vi "RIOduino Periodic.vi"   [LabVIEW 2015]
uses:
  <vilib>/Rock Robotics/SystemInterfaces/i2clib/i2c_bus.ctl
  <vilib>/Rock Robotics/Network Tables/NT Read Boolean.vi
  Global_Var/Drive_Global.vi
  Global_Var/JoyStick_Global.vi
types:
  T1 = typedef "WPI_DriverStationRobotMode2.ctl" = enum16{"Autonomous Disabled", "Autonomous Enabled", "Teleop Disabled", "Teleop Enabled", "Disconnected", "Finish", "Test Disabled", "Test Enabled", "Emergency Stopped"}
  T2 = typedef "WPI_DriverStationAllianceInfo.ctl" = enum16{"Red", "Blue", "Invalid"}
  T3 = typedef "WPI_I2CDevRef.ctl" = cluster{"DevStatus":errorcluster, "Device Address":u8, "Handle":i32, "I2C Bus":T4}
  T4 = typedef "i2c_bus.ctl" = enum16{"I2C On-Board", "I2C MXP", "Invalid"}
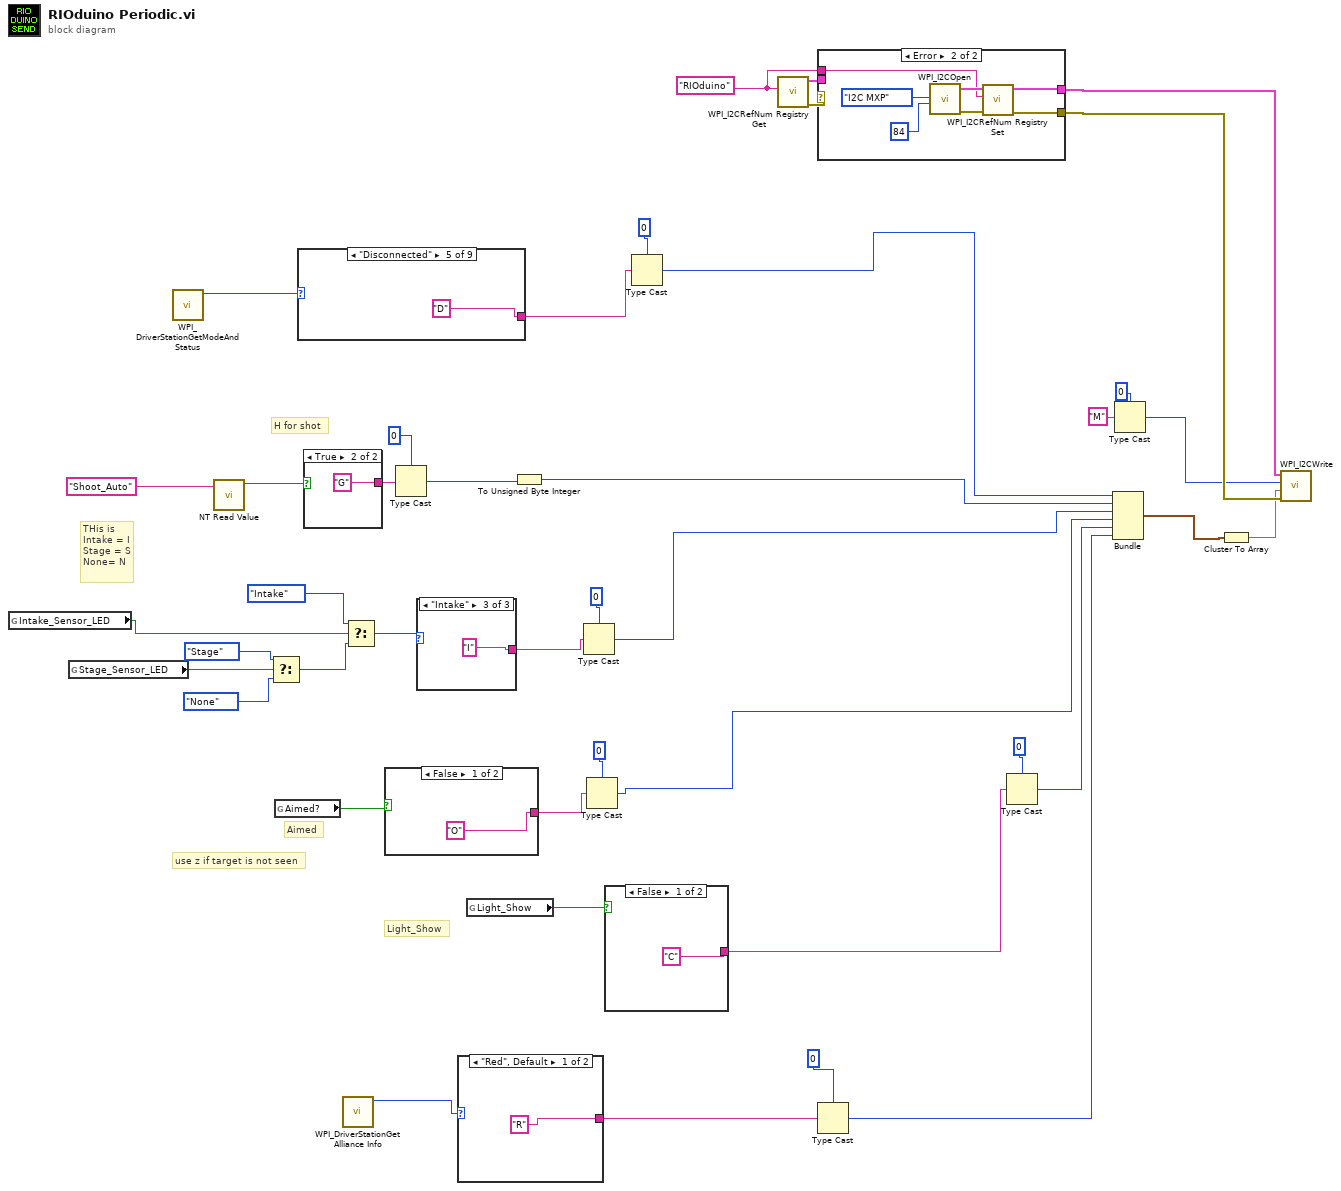
[diagram p0: block diagram]
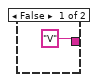
[diagram p2: hidden frame]
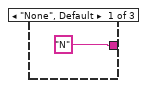
[diagram p3: hidden frame]
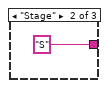
[diagram p4: hidden frame]
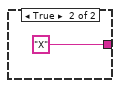
[diagram p5: hidden frame]
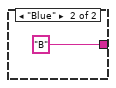
[diagram p6: hidden frame]
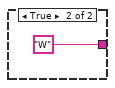
[diagram p7: hidden frame]
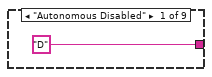
[diagram p8: hidden frame]
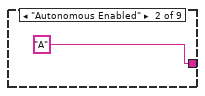
[diagram p9: hidden frame]
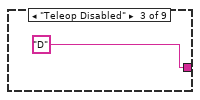
[diagram p10: hidden frame]
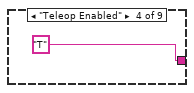
[diagram p11: hidden frame]
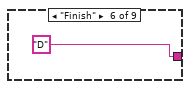
[diagram p12: hidden frame]
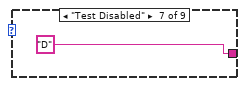
[diagram p13: hidden frame]
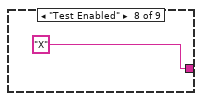
[diagram p14: hidden frame]
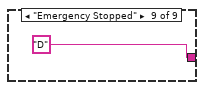
[diagram p15: hidden frame]
diagram:
  w40 = "RIOduino" ("refnum name")
  # "use z if target is not seen"
  # "H for shot"
  # "Light_Show"
  # "Aimed"
  # "THis is \nIntake = I\nStage = S\nNone= N"
  n1 = global read "JoyStick_Global.vi" "Intake_Sensor_LED"() -> (w5:bool)
  n2 = global read "JoyStick_Global.vi" "Stage_Sensor_LED"() -> (w9:bool)
  n3 = call <vilib>:"WPI_DriverStationGetModeAndStatus.vi"() -> ("Robot Mode"=w34:T1)  [unwired: 10 in, 1 out]
  n4 = call-poly <vilib>:"NT Read Value.vi"("Name"="Shoot_Auto") -> ("Boolean"=w1:bool)  [unwired: 9 in, 1 out]
  n5 = Select(t=enum16{"None", "Stage", "Intake"}."Stage", s=w9, f=enum16{"None", "Stage", "Intake"}."None") -> (s? t:f=w6:enum16{"None", "Stage", "Intake"})
  n6 = global read "Drive_Global.vi" "Aimed?"() -> (w12:bool)
  n7 = case shown="\"Disconnected\"" w34 {
    tunnel: ["D" "A" "D" "T" "D" "D" "D" "X" "D"] -> w27
    frame "Autonomous Disabled" {
    }
    frame "Autonomous Enabled" {
    }
    frame "Teleop Disabled" {
    }
    frame "Teleop Enabled" {
    }
    frame "Disconnected" {
    }
    frame "Finish" {
    }
    frame "Test Disabled" {
    }
    frame "Test Enabled" {
    }
    frame "Emergency Stopped" {
    }
  }
  n8 = case shown="True" w1 {
    tunnel: ["V" "G"] -> w17
    frame False {
    }
    frame True {
    }
  }
  n9 = call <vilib>:"WPI_DriverStationGet Alliance Info.vi"() -> ("Alliance"=w23:T2)  [unwired: 10 in, 1 out]
  n10 = Select(t=enum16{"None", "Stage", "Intake"}."Intake", s=w5, f=w6) -> (s? t:f=w4:enum16{"None", "Stage", "Intake"})
  n11 = case shown="False" w12 {
    tunnel: ["O" "X"] -> w14
    frame False {
    }
    frame True {
    }
  }
  n12 = Type Cast(type=u8 0, x=w17) -> (*(type *) &x=w18:u8)
  n13 = case shown="\"Intake\"" w4 {
    tunnel: ["N" "S" "I"] -> w3
    frame "None", Default {
    }
    frame "Stage" {
    }
    frame "Intake" {
    }
  }
  n14 = case shown="\"Red\", Default" w23 {
    tunnel: ["R" "B"] -> w21
    frame "Red", Default {
    }
    frame "Blue" {
    }
  }
  n15 = global read "JoyStick_Global.vi" "Light_Show"() -> (w11:bool)
  n16 = To Unsigned Byte Integer(number=w18) -> (unsigned 8bit integer=w33:u8)
  n17 = Type Cast(type=u8 0, x=w3) -> (*(type *) &x=w29:u8)
  n18 = Type Cast(type=u8 0, x=w14) -> (*(type *) &x=w15:u8)
  n19 = case shown="False" w11 {
    tunnel: ["C" "W"] -> w24
    frame False {
    }
    frame True {
    }
  }
  n20 = Type Cast(type=u8 0, x=w27) -> (*(type *) &x=w26:u8)
  n21 = call <vilib>:"WPI_I2CRefNum Registry Get.vi"("refnum name"=w40) -> ("error out"=w38:errorcluster, "I2CDevRef"=w39:T3)  [unwired: 9 in]
  n22 = case shown="Error" w38 {
    selector: w38 -> [w64 _]
    tunnel: [w64 w66] -> w42
    tunnel: [w63 w67] -> w41
    tunnel: w39 -> [w63 _]
    tunnel: w40 -> [_ w65]
    frame No Error {
    }
    frame Error {
      n23 = call <vilib>:"WPI_I2COpen.vi"("Device Address"=u8 84, "I2C Bus"=i2c_bus."I2C MXP") -> ("error out"=w69:errorcluster, "I2CDevRef"=w68:T3)  [unwired: 8 in]
      n24 = call <vilib>:"WPI_I2CRefNum Registry Set.vi"("error in (no error)"=w69, "refnum name"=w65, "I2CDevRef"=w68) -> ("error out"=w66:errorcluster, "I2CDevRef"=w67:T3)  [unwired: 7 in]
    }
  }
  n25 = Type Cast(type=u8 0, x=w21) -> (*(type *) &x=w20:u8)
  n26 = Type Cast(type=u8 0, x=w24) -> (*(type *) &x=w32:u8)
  n27 = Bundle(w26, w33, w29, w15, w32, w20) -> (w13:cluster{u8, u8, u8, u8, u8, u8})  [unwired: 1 in]
  n28 = Type Cast(type=u8 0, x="M") -> (*(type *) &x=w35:u8)
  n29 = Cluster To Array(cluster=w13) -> (array=w25:u8[])
  n30 = call <vilib>:"WPI_I2CWrite.vi"("error in (no error)"=w42, "I2CDataToSend"=w25, "I2CRegister"=w35, "I2CDevRef"=w41) -> ()  [unwired: 6 in, 2 out]
